vi "main.vi"() -> ()   [LabVIEW 2018]
doc: "Program służy do mierzenia napięć na wejściu i wyjściu czwórników."
uses:
  Control 1.ctl
panel:
  out "XY Graph":cluster{dbl[], "częstotliwość":dbl[]}(graph)
  out "U_Wy[tab]":dbl[](array[numeric])
  out "U_we[tab]":dbl[](array[numeric])
  in  "Wykres Y":u16(ring) items=["lin", "log"]
  in  "Wykres X":u16(ring) items=["lin", "log"]
  out "częstotliwość":dbl[](array[numeric])
  in  "Częstotliwość górna pomiaru [Hz]":dbl=100000.0 min=0.0001 max=130000.0 step=0.0001
  in  "save":bool
  in  "Częstotliwość dolna pomiaru [Hz]":dbl=5.0 min=0.0001 max=130000.0 step=0.0001
  in  "Przerwij":bool
  in  "Ilość punktów pomiaru":u32=10 min=1 step=1
  in  "Kanał":u16(ring)=1 items=["Ch1"=1, "Ch2"=2, "Ch3"=3, "Ch4"=4]
  in  "Rozłożenie punktów":u16(ring) items=["lin", "log"]
  in  "Amplituda [mV]":dbl=0.001 min=0.001 max=9999.9 step=0.001
  in  "Cancel":bool
  in  "połącz multimetr":bool
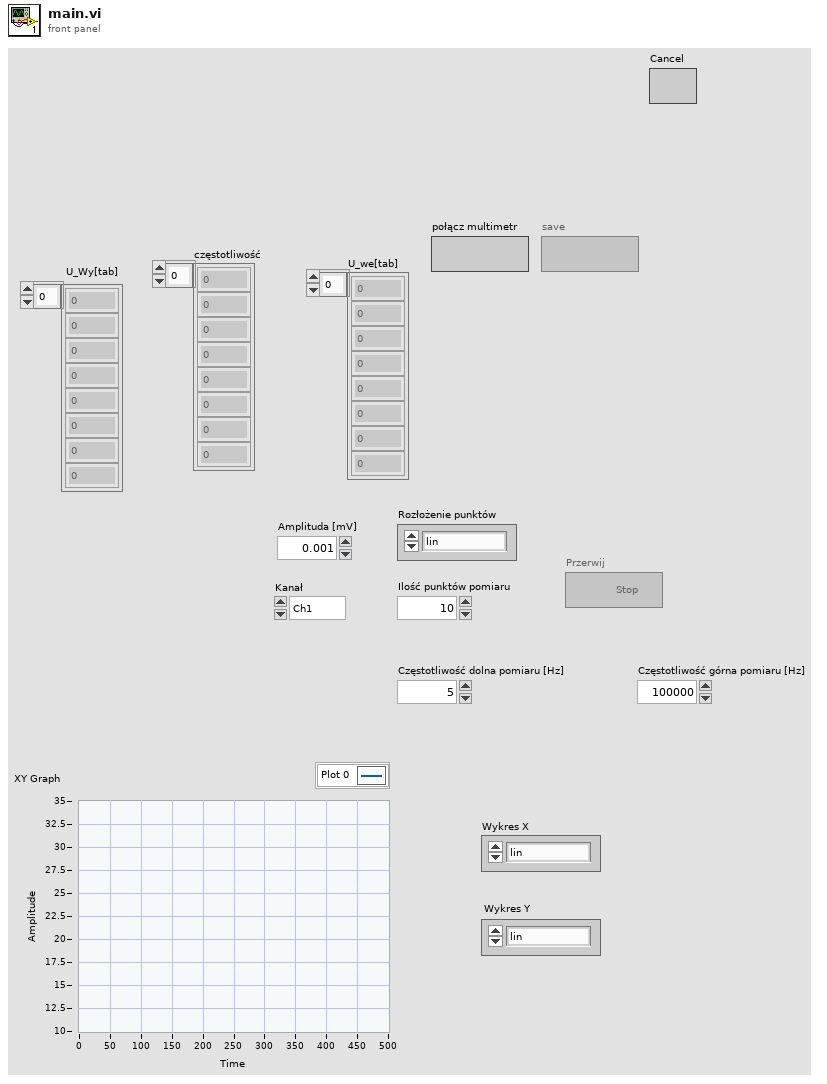
[diagram p1: front panel]
types:
  T1 = typedef "Control 1.ctl" = enum16{"convert", "draw", "init", "idle", "stop", "measure", "save"}
  T2 = enum8{"Enabled", "Disabled", "Disabled and Grayed Out"}
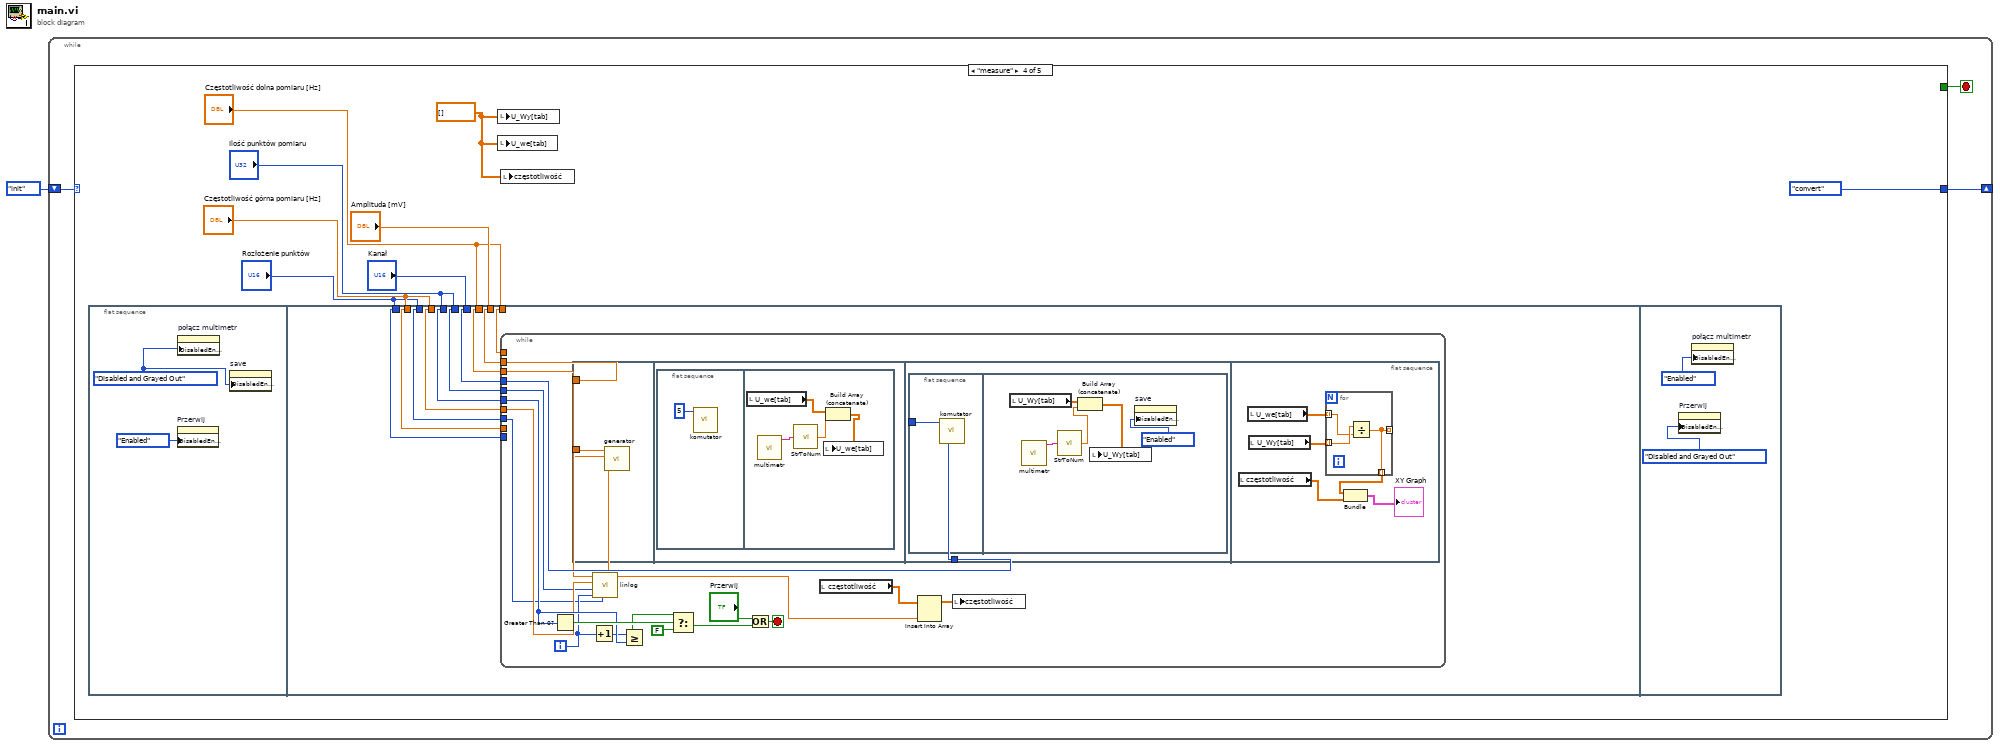
[diagram p0: block diagram]
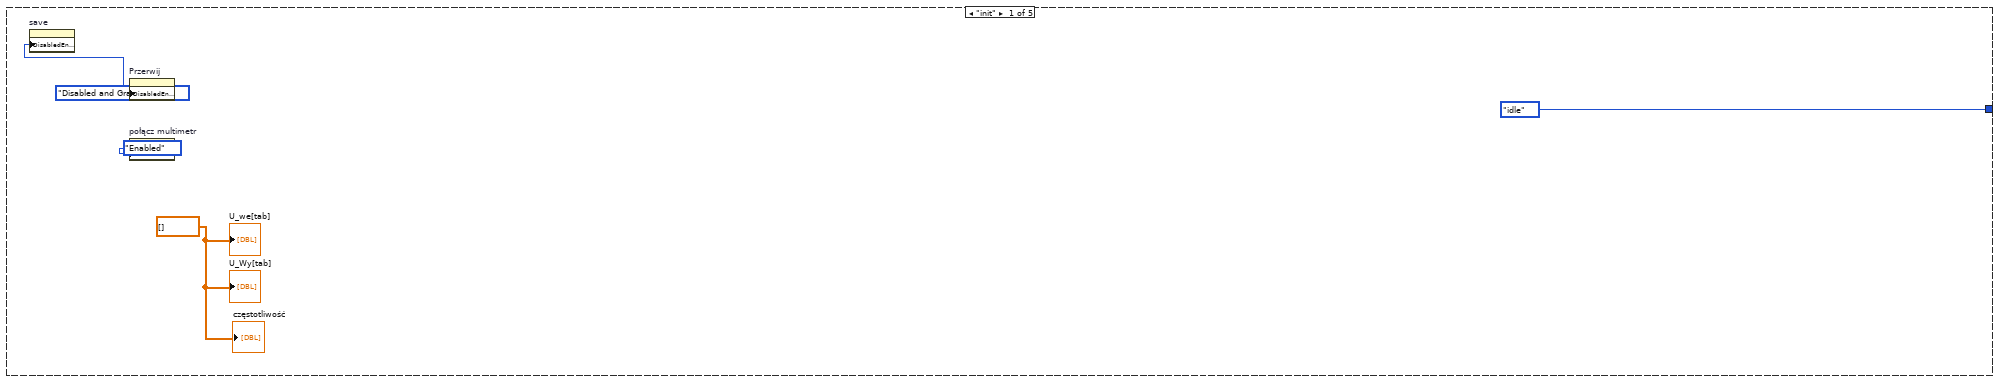
[diagram p2: hidden frame]
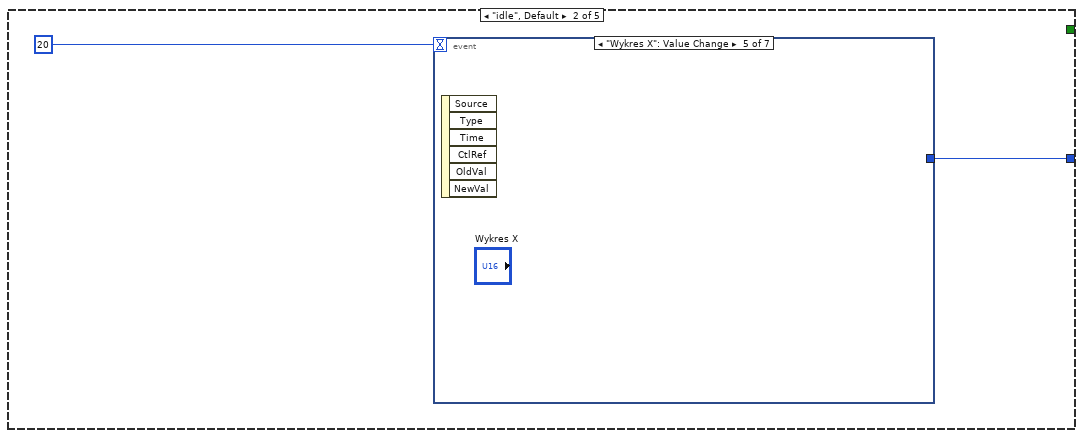
[diagram p3: hidden frame]
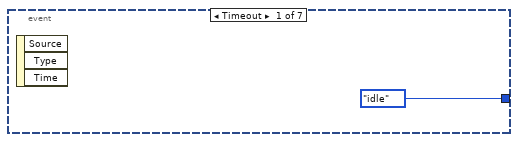
[diagram p4: hidden frame]
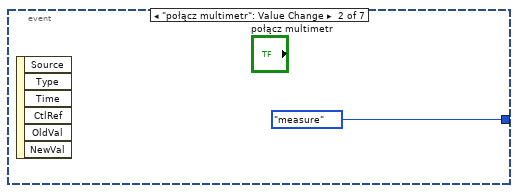
[diagram p5: hidden frame]
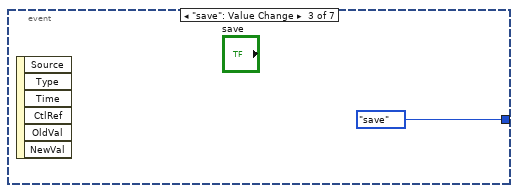
[diagram p6: hidden frame]
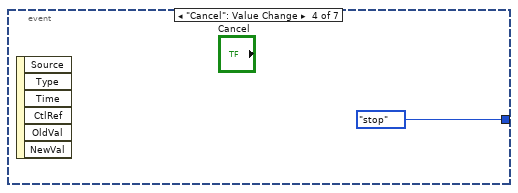
[diagram p7: hidden frame]
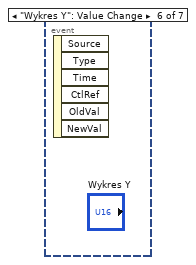
[diagram p8: hidden frame]
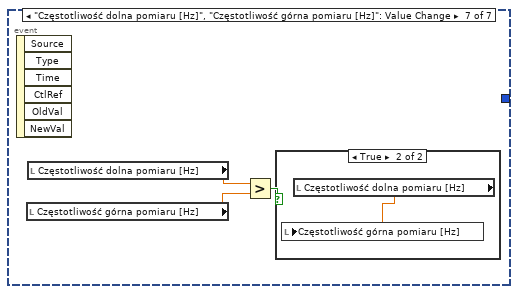
[diagram p9: hidden frame]
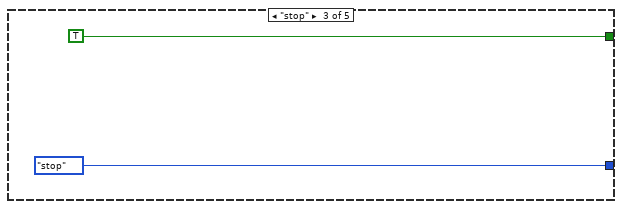
[diagram p11: hidden frame]
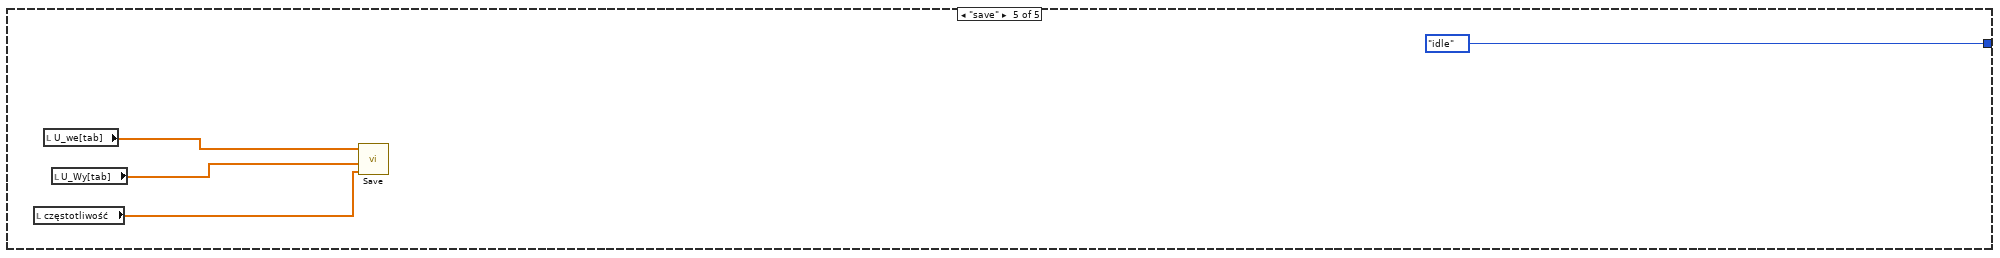
[diagram p12: hidden frame]
diagram:
  n1 = while {
    shift-right: [w2] -> _
    shift-left: Control_1."init" -> [w4]
    stop <- w3 stop-if-true
    n2 = case shown="\"measure\"" w4 {
      tunnel: [_ _ TRUE _ _] -> w3
      tunnel: [Control_1."idle" w9 Control_1."stop" Control_1."convert" Control_1."idle"] -> w2
      frame "init" {
        w5 = dbl[] []
        w6 = T2."Disabled and Grayed Out" ("Disabled")
        n3 = property on="save" class="Bool"("DisabledEnum"=w6) -> ()  [unwired: 2 in, 2 out]
        n4 = property on="Przerwij" class="Bool"("DisabledEnum"=w6) -> ()  [unwired: 2 in, 2 out]
        n5 = property on="połącz multimetr" class="Bool"("DisabledEnum"=T2."Enabled" ("Disabled")) -> ()  [unwired: 2 in, 2 out]
        "U_we[tab]" <- w5
        "U_Wy[tab]" <- w5
        "częstotliwość" <- w5
      }
      frame "idle", Default {
        n6 = event shown="[4] \"Wykres X\": Value Change" {
          selector: _ -> [_ _ _ _ _ _ _]
          dyn-events: _ -> [_ _ _ _ _ _ _]
          timeout: 20 -> [_ _ _ _ _ _ _]
          tunnel: [Control_1."idle" Control_1."measure" Control_1."save" Control_1."stop" _ _ _] -> w9
          event Timeout {
            n7 = event-data() -> ()  [unwired: 1 in, 3 out]
          }
          event "połącz multimetr": Value Change {
            n8 = event-data() -> ()  [unwired: 1 in, 6 out]
          }
          event "save": Value Change {
            n9 = event-data() -> ()  [unwired: 1 in, 6 out]
          }
          event "Cancel": Value Change {
            n10 = event-data() -> ()  [unwired: 1 in, 6 out]
          }
          event "Wykres X": Value Change {
            n11 = event-data() -> ()  [unwired: 1 in, 6 out]
          }
          event "Wykres Y": Value Change {
            n12 = event-data() -> ()  [unwired: 1 in, 6 out]
          }
          event "Częstotliwość dolna pomiaru [Hz]", "Częstotliwość górna pomiaru [Hz]": Value Change {
            n13 = event-data() -> ()  [unwired: 1 in, 6 out]
            n14 = local read "Częstotliwość górna pomiaru [Hz]"() -> (w16:dbl)
            n15 = local read "Częstotliwość dolna pomiaru [Hz]"() -> (w17:dbl)
            n16 = Greater?(x=w17, y=w16) -> (0:w15:bool)
            n17 = case shown="True" w15 {
              frame False {
              }
              frame True {
                n18 = local read "Częstotliwość dolna pomiaru [Hz]"() -> (w18:dbl)
                n19 = local write "Częstotliwość górna pomiaru [Hz]"(w18) -> ()
              }
            }
          }
        }
      }
      frame "stop" {
      }
      frame "measure" {
        w21 = dbl[] []
        n20 = flat-sequence {
          tunnel: "Ilość punktów pomiaru" -> [w40]
          tunnel: "Rozłożenie punktów" -> [w39]
          tunnel: "Kanał" -> [w38]
          tunnel: "Amplituda [mV]" -> [w37]
          tunnel: "Częstotliwość górna pomiaru [Hz]" -> [w36]
          tunnel: "Częstotliwość dolna pomiaru [Hz]" -> [w35]
          tunnel: "Częstotliwość dolna pomiaru [Hz]" -> [w34]
          tunnel: "Częstotliwość górna pomiaru [Hz]" -> [w33]
          tunnel: "Ilość punktów pomiaru" -> [w32]
          tunnel: "Rozłożenie punktów" -> [w31]
          frame #0 {
            w29 = T2."Disabled and Grayed Out" ("Disabled")
            n21 = property on="Przerwij" class="Bool"("DisabledEnum"=T2."Enabled" ("Disabled")) -> ()  [unwired: 2 in, 2 out]
            n22 = property on="połącz multimetr" class="Bool"("DisabledEnum"=w29) -> ()  [unwired: 2 in, 2 out]
            n23 = property on="save" class="Bool"("DisabledEnum"=w29) -> ()  [unwired: 2 in, 2 out]
          }
          frame #1 {
            n24 = while {
              tunnel: w40 -> [w57]
              tunnel: w39 -> [_]
              tunnel: w38 -> [w52]
              tunnel: w37 -> [w49]
              tunnel: w36 -> [_]
              tunnel: w35 -> [_]
              tunnel: w34 -> [w48]
              tunnel: w33 -> [w47]
              tunnel: w32 -> [w46]
              tunnel: w31 -> [w44]
              i -> [w45]
              stop <- w56 stop-if-true
              n25 = Greater Than 0?(x=w57) -> (x > 0?=w58:bool)
              n26 = flat-sequence {
                tunnel: w49 -> [w60]
                tunnel: w42 -> [w59]
                tunnel: w52 -> [w66]
                frame #0 {
                  n27 = call "generator.vi"("amplituda"=w60, "częstotliwość"=w59) -> ()  [unwired: 9 in, 1 out]
                }
                frame #1 {
                  n28 = flat-sequence {
                    frame #0 {
                      n29 = call "komutator.vi"("Numeric"=5) -> ()  [unwired: 11 in]
                    }
                    frame #1 {
                      n30 = local read "U_we[tab]"() -> (w65:dbl[])
                      n31 = call "multimetr.vi"() -> ("read buffer"=w64:string)  [unwired: 11 in]
                      n32 = call "StrToNum.vi"("String"=w64) -> ("number"=w63:dbl)
                      n33 = Build Array (concatenate)(w65, w63) -> (w62:dbl[])
                      n34 = local write "U_we[tab]"(w62) -> ()
                    }
                  }
                }
                frame #2 {
                  n35 = flat-sequence {
                    tunnel: w66 -> [w67]
                    frame #0 {
                      n36 = call "komutator.vi"("Numeric"=w67) -> ()  [unwired: 11 in]
                    }
                    frame #1 {
                      n37 = local read "U_Wy[tab]"() -> (w71:dbl[])
                      n38 = call "multimetr.vi"() -> ("read buffer"=w72:string)  [unwired: 11 in]
                      n39 = call "StrToNum.vi"("String"=w72) -> ("number"=w70:dbl)
                      n40 = Build Array (concatenate)(w71, w70) -> (w69:dbl[])
                      n41 = local write "U_Wy[tab]"(w69) -> ()
                      n42 = property on="save" class="Bool"("DisabledEnum"=T2."Enabled" ("Disabled")) -> ()  [unwired: 2 in, 2 out]
                    }
                  }
                }
                frame #3 {
                  n43 = local read "częstotliwość"() -> (w75:dbl[])
                  n44 = local read "U_we[tab]"() -> (w77:dbl[])
                  n45 = local read "U_Wy[tab]"() -> (w76:dbl[])
                  n46 = for {
                    tunnel: w77 -> [w79] mode=indexing
                    tunnel: w76 -> [w80] mode=indexing
                    tunnel: [w78] -> _ mode=indexing
                    tunnel: [w78] -> w74 mode=indexing
                    n47 = Divide(x=w80, y=w79) -> (x/y=w78:dbl)
                  }
                  n48 = Bundle(w74, "częstotliwość"=w75) -> (→"XY Graph":cluster{dbl[], "częstotliwość":dbl[]})  [unwired: 1 in]
                }
              }
              n49 = Increment(x=w45) -> (x+1=w51:i32)
              n50 = call "linlog.vi"("CzyLog"=w44, "Iteracja"=w45, "pkt"=w46, "max"=w47, "min"=w48) -> ("częstotliwość"=w42:dbl)  [unwired: 6 in]
              n51 = Greater Or Equal?(x=w51, y=w57) -> (x >= y?=w54:bool)
              n52 = Select(t=w54, s=w58, f=FALSE) -> (s? t:f=w53:bool)
              n53 = Or(x="Przerwij", y=w53) -> (x .or. y?=w56:bool)
              n54 = local read "częstotliwość"() -> (w43:dbl[])
              n55 = Insert Into Array(array=w43, new element=w42) -> (w41:dbl[])  [unwired: 1 in]
              n56 = local write "częstotliwość"(w41) -> ()
            }
          }
          frame #2 {
            n57 = property on="Przerwij" class="Bool"("DisabledEnum"=T2."Disabled and Grayed Out" ("Disabled")) -> ()  [unwired: 2 in, 2 out]
            n58 = property on="połącz multimetr" class="Bool"("DisabledEnum"=T2."Enabled" ("Disabled")) -> ()  [unwired: 2 in, 2 out]
          }
        }
        n59 = local write "U_Wy[tab]"(w21) -> ()
        n60 = local write "U_we[tab]"(w21) -> ()
        n61 = local write "częstotliwość"(w21) -> ()
      }
      frame "save" {
        n62 = local read "częstotliwość"() -> (w83:dbl[])
        n63 = local read "U_we[tab]"() -> (w85:dbl[])
        n64 = local read "U_Wy[tab]"() -> (w84:dbl[])
        n65 = call "Save.vi"("częstotliwość"=w83, "Wartosci na wyjsciu"=w84, "Wartosci na wejsciu"=w85) -> ()  [unwired: 9 in]
      }
    }
  }
